vi "event.vi"(8 "type":string, 9 "da ta":string[](array[string]), 10 "status":bool, 11 "eventid":dbl) -> (1 "output cluster":T1)   [LabVIEW 2023]
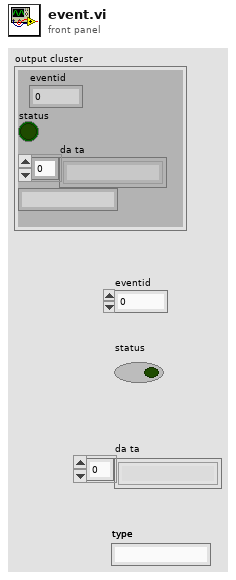
[diagram p1: front panel]
types:
  T1 = cluster{"eventid":dbl, "status":bool, "da ta":string[], string}
  T2 = cluster{"eventid":dbl, "status":bool, "da ta":string[], "type":string}
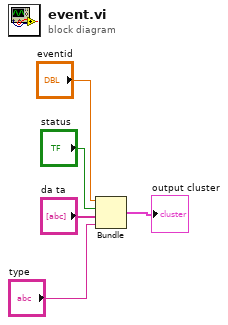
[diagram p0: block diagram]
diagram:
  n1 = Bundle("eventid"="eventid", "status"="status", "da ta"="da ta", "type"="type") -> (→"output cluster":T2)  [unwired: 1 in]
